vi "mass_flow_rate_element.vi"(1 "Density [g/cm3]":dbl, 2 "dP [Pa]":dbl) -> (0 "Mass Flow Rate [g/s]":dbl)   [LabVIEW 2017]
uses:
  Sensor Translation/sensor_translation.lvlib
  Sensor Translation/pressure_unit_converter.vi
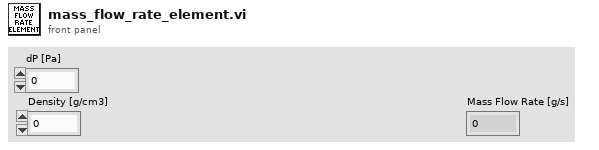
[diagram p1: front panel]
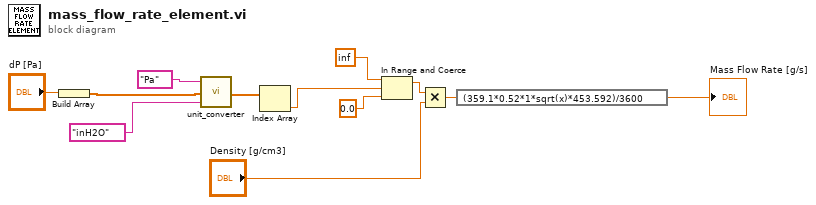
[diagram p0: block diagram]
diagram:
  n1 = Build Array("dP [Pa]") -> (w3:dbl[])
  n2 = call-poly "unit_converter.vi"("Output Unit"="inH2O", "Input"=w3, "Input Unit"="Pa") -> ("Output"=w2:dbl[])
  n3 = Index Array(array=w2) -> (element=w1:dbl)  [unwired: 1 in]
  n4 = In Range and Coerce(upper limit=inf, x=w1, lower limit=0.0 ("upper limit")) -> (coerced(x)=w7:dbl)  [unwired: 1 out]
  n5 = Multiply(x=w7, y="Density [g/cm3]") -> (x*y=w11:dbl)
  n6 = expression code="(359.1*0.52*1*sqrt(x)*453.592)/3600"(w11) -> (→"Mass Flow Rate [g/s]":dbl)
